vi "AWS S3 ls.vi"(8 "error in (no error)":errorcluster, 9 "prefix":string, 10 "bucket":string, 11 "LV-Data.AWS CLI in":refnum<class "LV-Data.AWS CLI.lvclass">) -> (0 "error out":errorcluster, 2 "Array Output":string[](array[string]), 3 "LV-Data.AWS CLI out":refnum<class "LV-Data.AWS CLI.lvclass">)   [LabVIEW 2019, in "LV-Data.AWS CLI.lvclass"]
uses:
  LV-Data.AWS CLI.lvclass
  LV-Data.AWS CLI.lvclass/LV-Data.AWS CLI.ctl
  <vilib>/AWS Toolkit/S3/Storage Class.ctl
  <vilib>/AWS Toolkit/S3/NI_AWS_S3.lvlib
  <vilib>/AWS Toolkit/S3/Owner.ctl
  <vilib>/AWS Toolkit/S3/Object Content.ctl
panel:
  out "std out":string
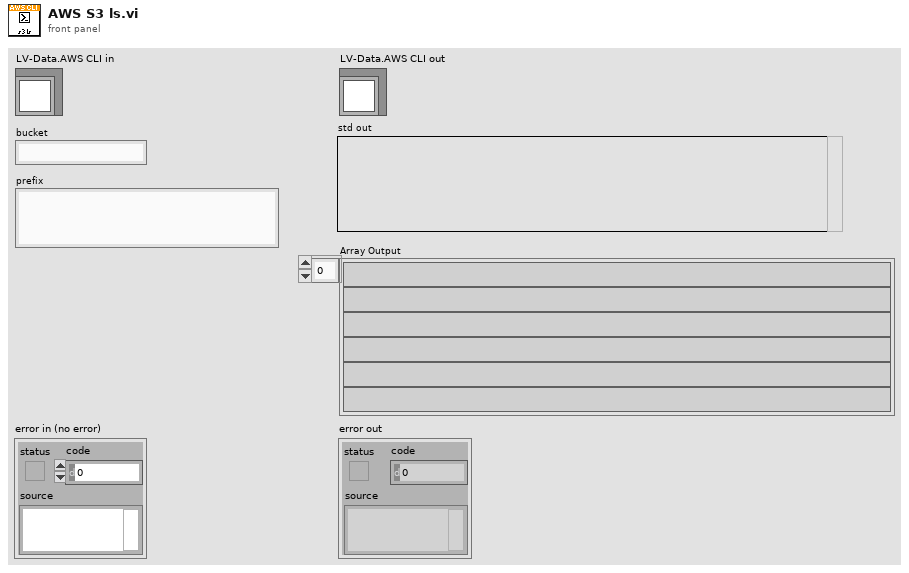
[diagram p1: front panel]
types:
  T1 = typedef "NI_AWS_S3.lvlib/Object Content.ctl" = cluster{"Key":string, "Last Modified":timestamp, "ETag":string, "Size":u64, "Storage Class":T2, "Owner":T3}
  T2 = typedef "NI_AWS_S3.lvlib/Storage Class.ctl" = enum16{"STANDARD", "REDUCED_REDUNDANCY"}
  T3 = typedef "NI_AWS_S3.lvlib/Owner.ctl" = cluster{"ID":string, "Display Name":string}
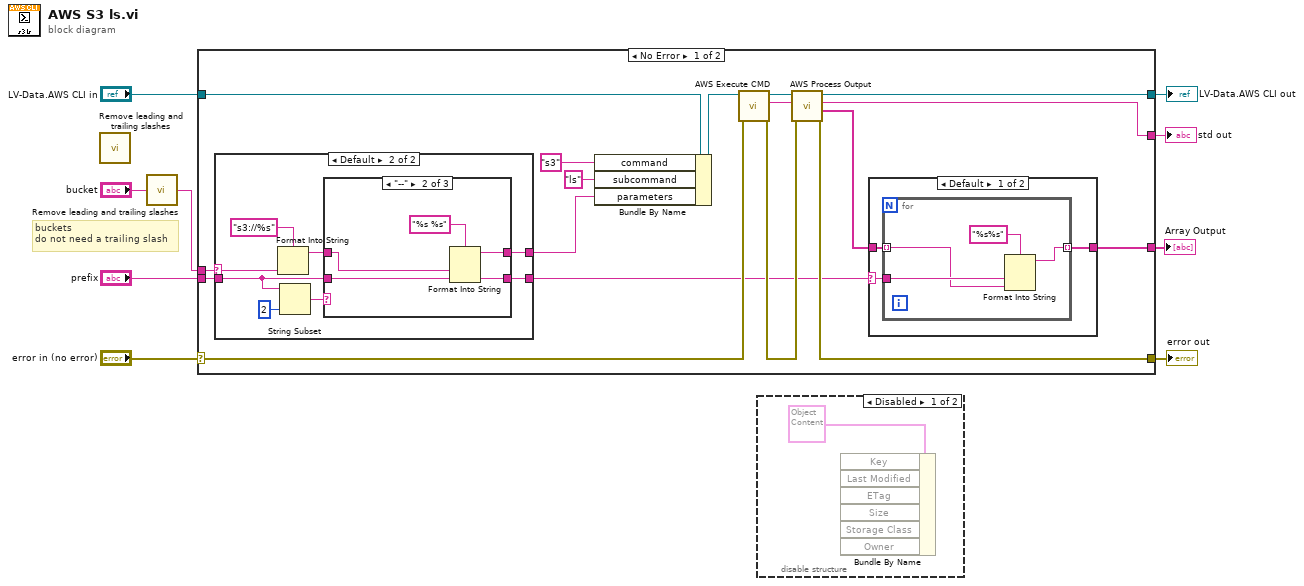
[diagram p0: block diagram]
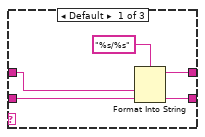
[diagram p4: hidden frame]
diagram:
  # "buckets\ndo not need a trailing slash"
  n1 = call "Remove leading and trailing slashes.vi"() -> ()  [unwired: 1 in, 1 out]
  n2 = call "Remove leading and trailing slashes.vi"("string in"="bucket") -> ("string out"=w3:string)
  n3 = case shown="No Error" "error in (no error)" {
    selector: "error in (no error)" -> [w26 w55]
    tunnel: [w13 w55] -> w8
    tunnel: [w17 w54] -> w6
    tunnel: "LV-Data.AWS CLI in" -> [w24 w54]
    tunnel: [w15 _] -> w5
    tunnel: w3 -> [w20 _]
    tunnel: "prefix" -> [w19 _]
    tunnel: [w11 _] -> w4
    frame No Error {
      n4 = case shown="Default" w20 {
        selector: w20 -> [_ w34]
        tunnel: [_ w33] -> w21
        tunnel: w19 -> [w27 w28]
        tunnel: [w27 w31] -> w12
        frame "" {
        }
        frame Default {
          n5 = Format Into String(format string="s3://%s", w34) -> (resulting string=w32:string)  [unwired: 2 in, 1 out]
          n6 = String Subset(string=w28, length (rest)=2 ("length (rest)")) -> (substring=w29:string)  [unwired: 1 in]
          n7 = case shown="\"--\"" w29 {
            selector: w29 -> [_ _ w44]
            tunnel: [w38 w42 w45] -> w33
            tunnel: w32 -> [w37 w41 w45]
            tunnel: [w36 w40 w44] -> w31
            tunnel: w28 -> [w36 w40 _]
            frame Default {
              n8 = Format Into String(format string="%s/%s", w37, w36) -> (resulting string=w38:string)  [unwired: 2 in, 1 out]
            }
            frame "--" {
              n9 = Format Into String(format string="%s %s", w41, w40) -> (resulting string=w42:string)  [unwired: 2 in, 1 out]
            }
            frame "" {
            }
          }
        }
      }
      n10 = Bundle By Name(cluster=w24, "command"="s3" ("CLI.command"), "subcommand"="ls" ("CLI.subcommand"), "parameters"=w21) -> (w25:refnum<class "LV-Data.AWS CLI.lvclass">)
      n11 = call "AWS Execute CMD.vi"("error in (no error)"=w26, "LV-Data.AWS CLI"=w25) -> ("error out"=w14:errorcluster, "std out"=w16:string, "LV-Data.AWS CLI out"=w18:refnum<class "LV-Data.AWS CLI.lvclass">)  [unwired: 7 in]
      n12 = call "AWS Process Output.vi"("error in"=w14, "standard output"=w16, "LV-Data.AWS CLI"=w18) -> ("error out"=w13:errorcluster, "Array Output"=w10:string[], "standard output"=w15:string, "LV-Data.AWS CLI out"=w17:refnum<class "LV-Data.AWS CLI.lvclass">)  [unwired: 5 in]
      n13 = case shown="Default" w12 {
        selector: w12 -> [w47 _]
        tunnel: [w48 w53] -> w11
        tunnel: w10 -> [w46 w53]
        frame Default {
          n14 = for {
            tunnel: [w51] -> w48 mode=indexing
            tunnel: w47 -> [w50]
            tunnel: w46 -> [w49] mode=indexing
            n15 = Format Into String(format string="%s%s", w50, w49) -> (resulting string=w51:string)  [unwired: 2 in, 1 out]
          }
        }
        frame "" {
        }
      }
    }
    frame Error {
    }
  }
  "error out" <- w8
  "LV-Data.AWS CLI out" <- w6
  "std out" <- w5
  "Array Output" <- w4
  n16 = disable-structure shown="Disabled" {
    frame Disabled {
      n17 = Bundle By Name(cluster=T1 {"Key"="", "Last Modified"=timestamp(0 s since 1904-01-01), "ETag"="", "Size"=0, "Storage Class"=enum."STANDARD", "Owner"={"ID"="", "Display Name"=""}} ("Content")) -> ()  [unwired: 6 in, 1 out]
    }
    frame Enabled {
    }
  }
